vi "Turning control.vi"(9 "Robot angle":dbl, 10 "Angle to move to":dbl) -> (3 "Final Robot angle":dbl)   [LabVIEW 2015]
panel:
  out "Angle to move":dbl
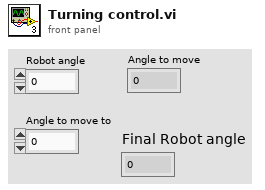
[diagram p1: front panel]
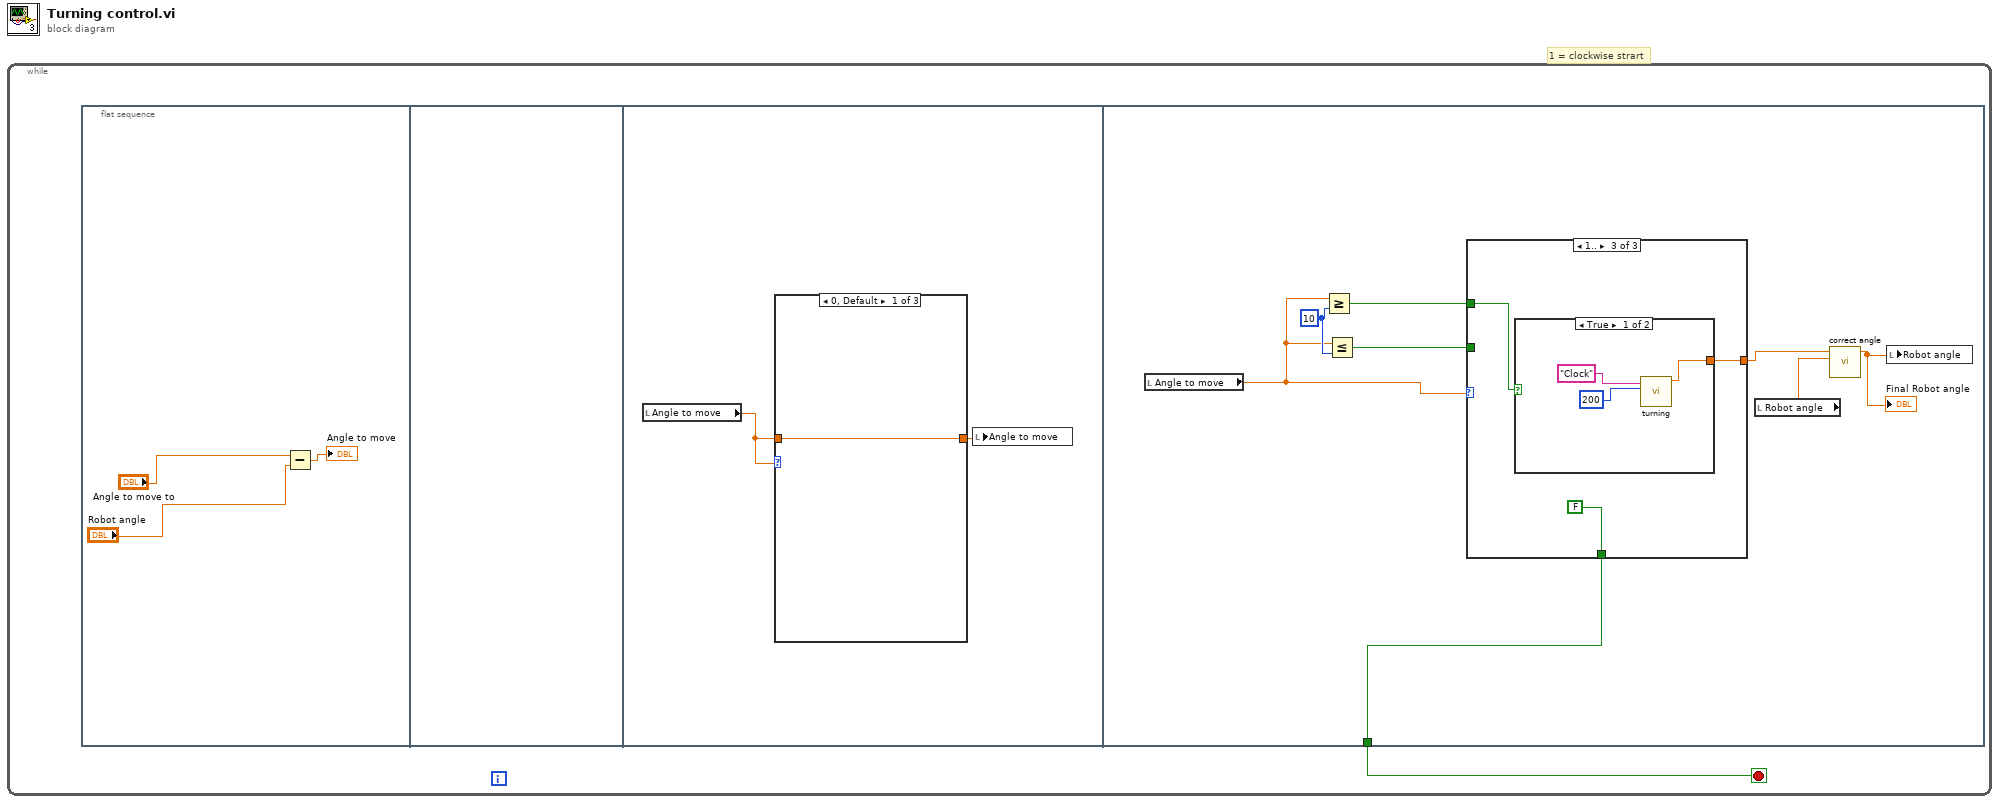
[diagram p0: block diagram]
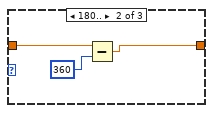
[diagram p2: hidden frame]
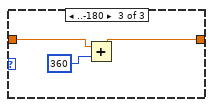
[diagram p3: hidden frame]
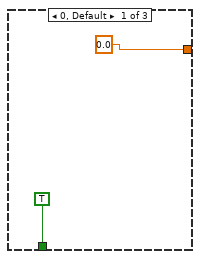
[diagram p4: hidden frame]
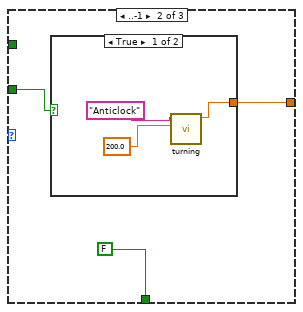
[diagram p5: hidden frame]
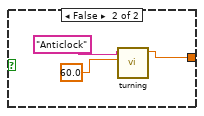
[diagram p6: hidden frame]
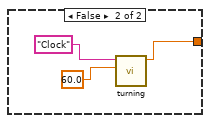
[diagram p7: hidden frame]
diagram:
  # "1 = clockwise strart"
  n1 = while {
    stop <- w1 stop-if-true
    n2 = flat-sequence {
      tunnel: [w21] -> w1
      frame #0 {
        n3 = Subtract(x="Angle to move to", y="Robot angle") -> (x-y=→"Angle to move":dbl)
      }
      frame #1 {
      }
      frame #2 {
        n4 = local read "Angle to move"() -> (w6:dbl)
        n5 = case shown="0, Default" w6 {
          tunnel: [w7 w10 w13] -> w5
          tunnel: w6 -> [w7 w8 w11]
          frame 0, Default {
          }
          frame 180.. {
            n6 = Subtract(x=w8, y=360) -> (x-y=w10:dbl)
          }
          frame ..-180 {
            n7 = Add(x=w11, y=360) -> (x+y=w13:dbl)
          }
        }
        n8 = local write "Angle to move"(w5) -> ()
      }
      frame #3 {
        w17 = 10
        n9 = local read "Angle to move"() -> (w16:dbl)
        n10 = Greater Or Equal?(x=w16, y=w17) -> (x >= y?=w15:bool)
        n11 = Less Or Equal?(x=w16, y=w17) -> (x <= y?=w14:bool)
        n12 = case shown="1.." w16 {
          tunnel: [TRUE FALSE FALSE] -> w21
          tunnel: [0.0 w25 w34] -> w20
          tunnel: w15 -> [_ _ w33]
          tunnel: w14 -> [_ w24 _]
          frame 0, Default {
          }
          frame ..-1 {
            n13 = case shown="True" w24 {
              tunnel: [w28 w31] -> w25
              frame True {
                n14 = call "turning.vi"("Turn time"=200.0, "clock anticlock"="Anticlock") -> ("angle moved"=w28:dbl)  [unwired: 9 in]
              }
              frame False {
                n15 = call "turning.vi"("Turn time"=60.0, "clock anticlock"="Anticlock") -> ("angle moved"=w31:dbl)  [unwired: 9 in]
              }
            }
          }
          frame 1.. {
            n16 = case shown="True" w33 {
              tunnel: [w37 w40] -> w34
              frame True {
                n17 = call "turning.vi"("Turn time"=200, "clock anticlock"="Clock") -> ("angle moved"=w37:dbl)  [unwired: 9 in]
              }
              frame False {
                n18 = call "turning.vi"("Turn time"=60.0, "clock anticlock"="Clock") -> ("angle moved"=w40:dbl)  [unwired: 9 in]
              }
            }
          }
        }
        n19 = local read "Robot angle"() -> (w19:dbl)
        n20 = call "correct angle.vi"("Robot angle"=w19, "Angle moved"=w20) -> ("Final angle"=w18:dbl)  [unwired: 9 in]
        "Final Robot angle" <- w18
        n21 = local write "Robot angle"(w18) -> ()
      }
    }
  }
